vi "Transform.vi"(8 "error in (no error)":errorcluster caption="entrée d'erreur (pas d'erreur)", 9 "y":string[][](array[string]), 10 "X":string[][](array[string]), 11 "FunctionTransformer.lvclass":refnum<class "FunctionTransformer.lvclass">) -> (0 "error in (no error)":errorcluster caption="entrée d'erreur (pas d'erreur)", 2 "Data":T1, 3 "FunctionTransformer.lvclass":refnum<class "FunctionTransformer.lvclass">)   [LabVIEW 2020, in "FunctionTransformer.lvclass"]
doc: "Transform X using the forward function.\n\nReturns : \n\n- X_out : char array-like, shape (n_samples, n_features)\n Transformed input."
uses:
  FunctionTransformer.lvclass
  FunctionTransformer.lvclass/FunctionTransformer.ctl
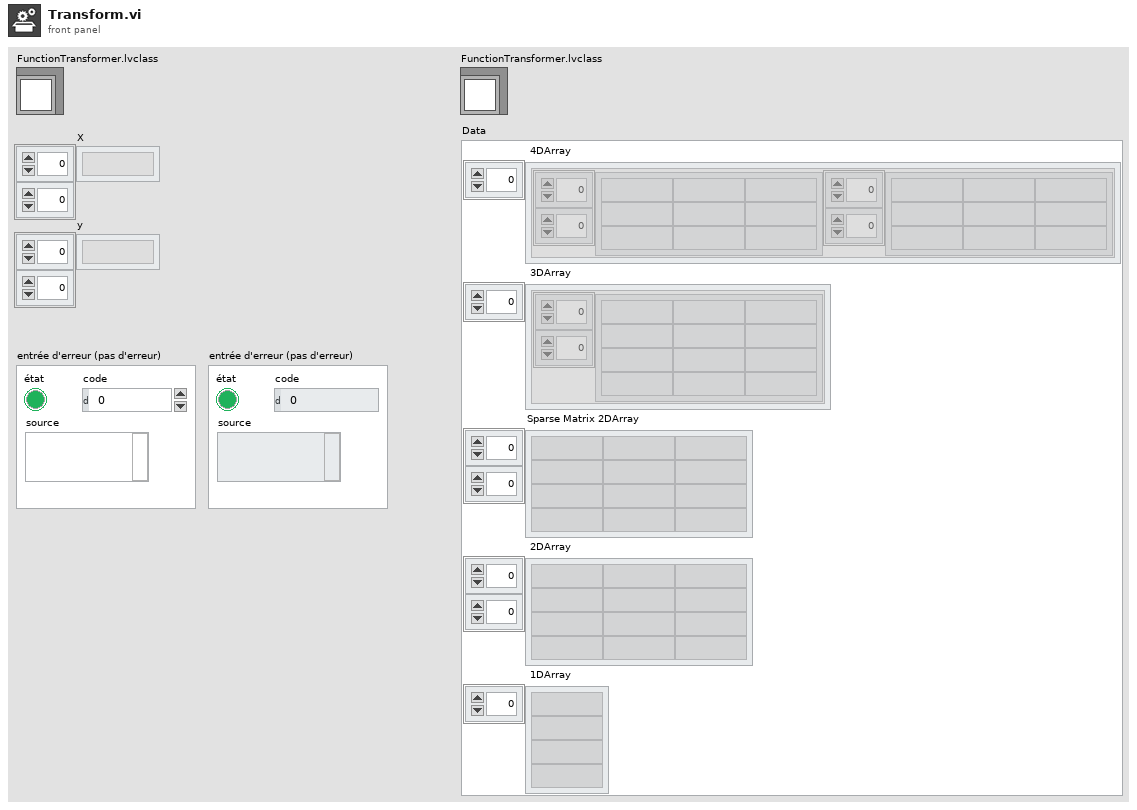
[diagram p1: front panel]
types:
  T1 = cluster{" 4DArray":cluster{"1":string[][], "2":string[][]}[], " 3DArray":cluster{"Tableau":string[][]}[], "Sparse Matrix 2DArray":string[][], " 2DArray":string[][], " 1DArray":string[]}
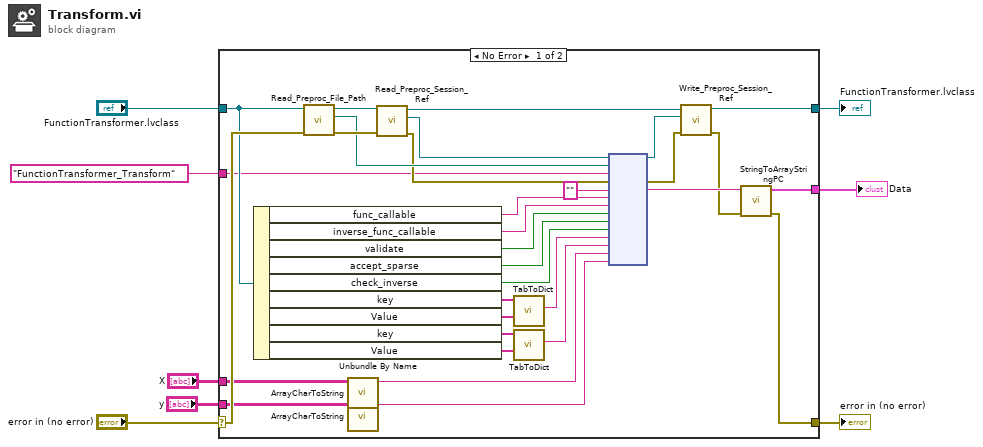
[diagram p0: block diagram]
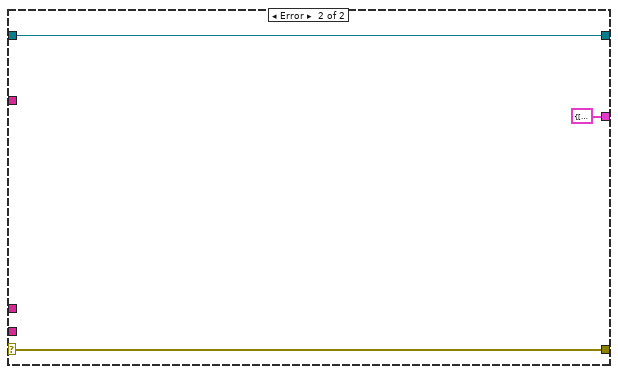
[diagram p2: hidden frame]
diagram:
  n1 = case shown="No Error" "error in (no error)" {
    selector: "error in (no error)" -> [w31 w43]
    tunnel: [w15 w43] -> w7
    tunnel: [w17 w42] -> w5
    tunnel: "FunctionTransformer.lvclass" -> [w30 w42]
    tunnel: "FunctionTransformer_Transform" ("Fonction") -> [w24 _]
    tunnel: [w18 T1 {" 4DArray"=[], " 3DArray"=[], "Sparse Matrix 2DArray"=[], " 2DArray"=[], " 1DArray"=[]} ("Data")] -> w1
    tunnel: "X" -> [w23 _]
    tunnel: "y" -> [w22 _]
    frame No Error {
      n2 = Unbundle By Name(w30) -> ("func_callable"=w29:string, "inverse_func_callable"=w28:string, "validate"=w27:bool, "accept_sparse"=w26:bool, "check_inverse"=w25:bool, "key"=w14:string[], "Value"=w13:string[], "key"=w11:string[], "Value"=w10:string[])
      n3 = call-dynamic "Read_Preproc_File_Path.vi"("error in (no error)"=w31, "Python in"=w30) -> ("error out"=w39:errorcluster, "File_Path"=w36:path, "Python out"=w40:refnum<class "FunctionTransformer.lvclass">)  [unwired: 7 in]
      n4 = call "ArrayCharToString.vi"("TAB"=w23) -> ("Instruction"=w21:string)  [unwired: 10 in]
      n5 = call "ArrayCharToString.vi"("TAB"=w22) -> ("Instruction"=w20:string)  [unwired: 10 in]
      n6 = call-dynamic "Read_Preproc_Session_Ref.vi"("error in (no error)"=w39, "Python in"=w40) -> ("error out"=w35:errorcluster, "Session_ref"=w37:refnum<k35>, "Python out"=w38:refnum<class "FunctionTransformer.lvclass">)  [unwired: 7 in]
      n7 = call "TabToDict.vi"("String Value"=w13, "String key"=w14) -> ("Dict with string value"=w12:string)  [unwired: 8 in, 1 out]
      n8 = call "TabToDict.vi"("String Value"=w10, "String key"=w11) -> ("Dict with string value"=w9:string)  [unwired: 8 in, 1 out]
      n9 = node(w37, w36, w24, w35, "", w29, w28, w27, w26, w25, w12, w9, w21, w20) -> (w33:refnum<k35>, w34:errorcluster, w19:string)  [unwired: 9 in, 2 out]
      n10 = call-dynamic "Write_Preproc_Session_Ref.vi"("error in (no error)"=w34, "Session_ref"=w33, "Python in"=w38) -> ("error out"=w16:errorcluster, "Python out"=w17:refnum<class "FunctionTransformer.lvclass">)  [unwired: 7 in]
      n11 = call "StringToArrayStringPC.vi"("sortie d'erreur"=w16, "Return value"=w19) -> ("sortie d'erreur"=w15:errorcluster, "Data"=w18:T1)  [unwired: 8 in]
    }
    frame Error {
    }
  }
  "error in (no error)" <- w7
  "FunctionTransformer.lvclass" <- w5
  "Data" <- w1
